vi "Calculate Next Zernike Vector.vi"(8 "error in (no error)":errorcluster) -> (0 "error out":errorcluster)   [LabVIEW 2015, in "Automation.lvlib"]
uses:
  Automation.lvlib
  Automation Loop State.ctl
  Camera/Acquisition Settings.ctl
  Camera/Camera.lvlib
  ZO Settings.ctl
  ZO State.ctl
  Automation State.ctl
  Zstack Settings.ctl
  Zstack State.ctl
panel:
  in  "Automation State in":T1={"Automation State"=enum."Idle", "Handle out"=0, "ZO State"={"ZO Settings"={"Acquisition Settings"={"Save?"=FALSE, "DCIMG Path"=path "", "Filename"="", "Total Frames"=0, "Sender"=enum."UI"}, "Shift Amplitude"=0.0, "Initial Zernike Vector"=[]}, "Zernike Size"=15, "Points per order"=15, "Zernike State"=enum."Idle", "Zernike Vectors"=[], "Total Frames"=15, "Current Frame"=15}, "Zstack State"={"Zstack Settings"={"Acquisition Settings"={"Save?"=FALSE, "DCIMG Path"=path "", "Filename"="", "Total Frames"=0, "Sender"=enum."UI"}, "XYZ start"=[], "XYZ end"=[]}, "Zstack State"=enum."Idle", "Stack Coordinates"=[], "Total Frames"=15, "Current Frame"=15}}
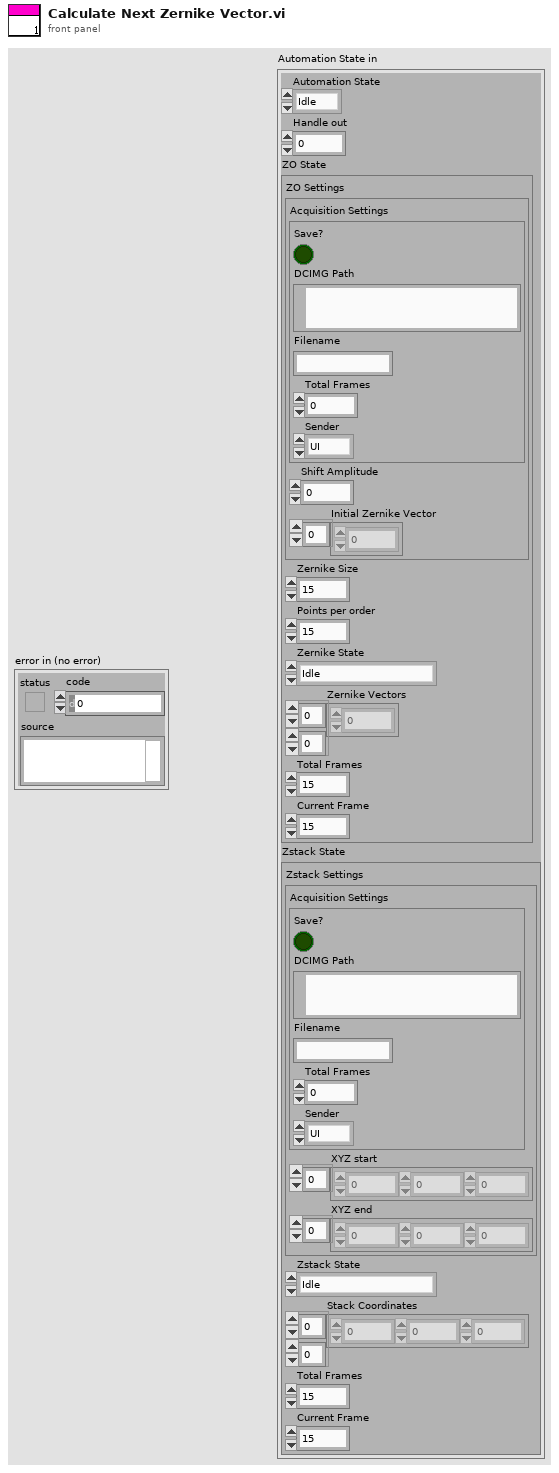
[diagram p1: front panel]
types:
  T1 = typedef "Automation.lvlib/Automation State.ctl" = cluster{"Automation State":T2, "Handle out":u32, "ZO State":T3, "Zstack State":T6}
  T2 = typedef "Automation.lvlib/Automation Loop State.ctl" = enum16{"Idle", "Zernike Optimization", "Z Stack"}
  T3 = typedef "Automation.lvlib/ZO State.ctl" = cluster{"ZO Settings":T4, "Zernike Size":i32, "Points per order":i32, "Zernike State":enum16{"Idle", "Waiting for Camera Init.", "Wait for camera frame", "Ready for new mirror config"}, "Zernike Vectors":dbl[][], "Total Frames":i32, "Current Frame":i32}
  T4 = typedef "Automation.lvlib/ZO Settings.ctl" = cluster{"Acquisition Settings":T5, "Shift Amplitude":dbl, "Initial Zernike Vector":dbl[]}
  T5 = typedef "Camera.lvlib/Acquisition Settings.ctl" = cluster{"Save?":bool, "DCIMG Path":path, "Filename":string, "Total Frames":i32, "Sender":enum16{"UI", "Automation"}}
  T6 = typedef "Automation.lvlib/Zstack State.ctl" = cluster{"Zstack Settings":T7, "Zstack State":enum16{"Idle", "Waiting for Camera Init.", "Wait for camera frame", "Ready for new position"}, "Stack Coordinates":dbl[][], "Total Frames":i32, "Current Frame":i32}
  T7 = typedef "Automation.lvlib/Zstack Settings.ctl" = cluster{"Acquisition Settings":T5, "XYZ start":dbl[], "XYZ end":dbl[]}
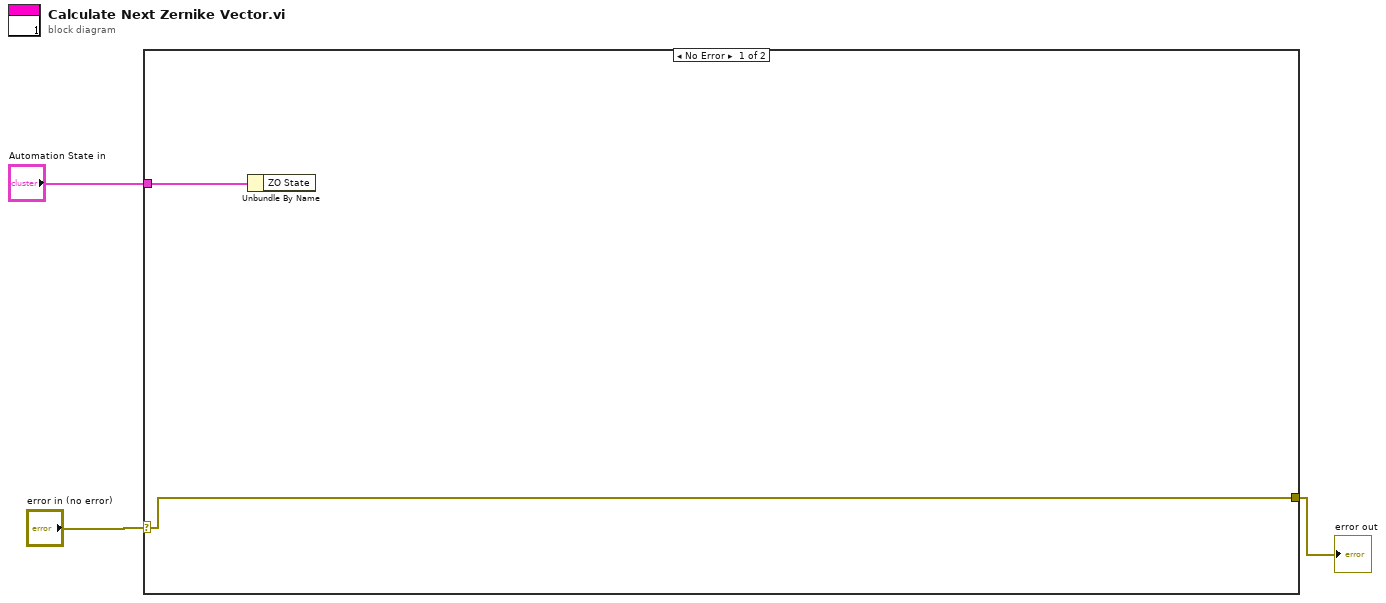
[diagram p0: block diagram]
diagram:
  n1 = case shown="No Error" "error in (no error)" {
    selector: "error in (no error)" -> [w6 w7]
    tunnel: [w6 w7] -> w2
    tunnel: "Automation State in" -> [w5 _]
    frame No Error {
      n2 = Unbundle By Name(w5) -> ("ZO State"=w4:T3)
    }
    frame Error {
    }
  }
  "error out" <- w2
